vi "Is Acquisition Done.vi"(0 "fpga interface in":refnum<k20>, 11 "error in (no error)":errorcluster) -> (4 "fpga interface out":refnum<k20>, 6 "acquisition done":bool, 15 "error out":errorcluster)   [LabVIEW 2023, in "GettingStarted_Acq_148X_Host.lvlib"]
uses:
  GettingStarted_Acq_148X_Host.lvlib
  Types/148x_Acq_FPGA_Reference.ctl
  <instrlib>/FlexRIO/CSI-2/v2/FPGA/Types/Global Acquisition Engine State.ctl
  <vilib>/Utility/error.llb/Error Cluster From Error Code.vi
  <vilib>/rvi/errors/niLvFpgaAdjustHostInterfaceError.vi
  <vilib>/rvi/interface/nirviReadWriteControl/nirviReadWriteControl.xnode
  <instrlib>/FlexRIO/CSI-2/v2/FPGA/NI CSI-2 API FPGA v2.lvlib
  NiFpgaLv.dll
  <vilib>/rvi/interface/Simulation/niFpgaSimulationCallBeginRW.vi
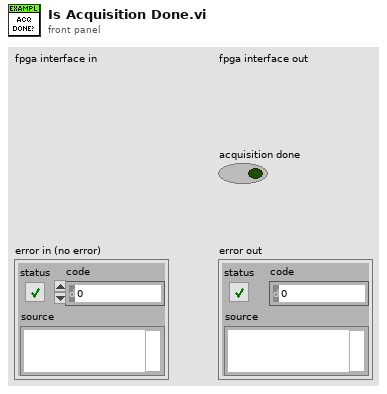
[diagram p1: front panel]
types:
  T1 = typedef "NI CSI-2 API FPGA v2.lvlib/Global Acquisition Engine State.ctl" = enum8{"Idle", "Ready For Start Trigger", "Acquire", "Error"}
  T2 = typedef "GettingStarted_Acq_148X_Host.lvlib/148x_Acq_FPGA_Reference.ctl" = refnum<k20>
  T3 = enum8{"Idle", "Ready For Start Trigger", "Acquire", "Error"}
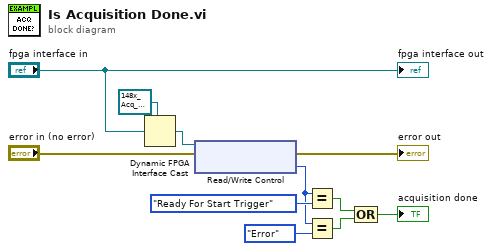
[diagram p0: block diagram]
diagram:
  n1 = Dynamic FPGA Interface Cast(Session In=T2 refnum ("FPGA VI Reference Out"), Type="fpga interface in") -> (Session Out=w8:T2)
  n2 = xnode "Read/Write Control"("FPGA VI Reference In"=w8, "error in"="error in (no error)") -> ("error out"=→"error out":errorcluster, "global acq state"=w4:T3)  [unwired: 1 out]
  n3 = Equal?(x=w4, y=Global_Acquisition_Engine_State."Ready For Start Trigger" ("element")) -> (x = y?=w2:bool)
  n4 = Equal?(x=w4, y=Global_Acquisition_Engine_State."Error" ("element")) -> (x = y?=w3:bool)
  n5 = Compound Arithmetic op=OR(w2, w3) -> (→"acquisition done":bool)
  "fpga interface out" <- "fpga interface in"
